vi "EMS Synchronize Status.vi"(8 "error in (no error)":errorcluster, 9 "Status":T1, 10 "error":string, 11 "Master Controller in":refnum<class "Master Controller.lvclass">) -> (0 "error out":errorcluster, 3 "Master Controller out":refnum<class "Master Controller.lvclass">)   [LabVIEW 2015, in "Master Controller Core.lvlib" / "Master Controller.lvclass"]
uses:
  Master Controller.lvclass
  SCADA Core/SCADA Abstract Messages/Simple Command Status Msg/Simple Command Status.ctl
  Communications/SCADA Communcations Actor/SCADA Communications/Controls/EMS Message Cluster.ctl
  Master Controller.lvclass/Master Controller.ctl
  Communications/SCADA Communcations Actor/SCADA Communications Messages/Transmit EMS Message Msg/Transmit EMS Message Msg.lvclass/Transmit EMS Message Msg.ctl
  <vilib>/ActorFramework/Message Enqueuer/Message Enqueuer.lvclass/Message Enqueuer.ctl
  <vilib>/ActorFramework/Message Enqueuer/Enqueue.vi
  <vilib>/ActorFramework/Message Priority Queue/Priority Enqueue.vi
  Communications/SCADA Communcations Actor/SCADA Communications Messages/Transmit EMS Message Msg/Transmit EMS Message Msg.lvclass
  Communications/SCADA Communcations Actor/SCADA Communications/SCADA Communications.lvclass
  Utilities/Message Strings.llb/Message String Utilities.lvlib
  Utilities/Status Messaging.llb/Status Messaging.lvlib
  SCADA Core/SCADA Abstract Messages/Simple Command Status Msg/Simple Command Status Msg.lvclass
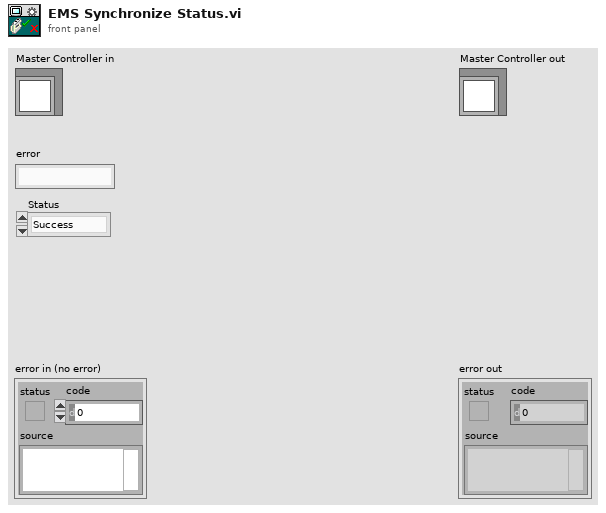
[diagram p1: front panel]
types:
  T1 = typedef "SCADA Core.lvlib/Simple Command Status Msg.lvclass/Simple Command Status.ctl" = enum16{"Success", "Failure"}
  T2 = typedef "SCADA Communcations Actor.lvlib/SCADA Communications.lvclass/EMS Message Cluster.ctl" = cluster{"Name":string, "Content":string}
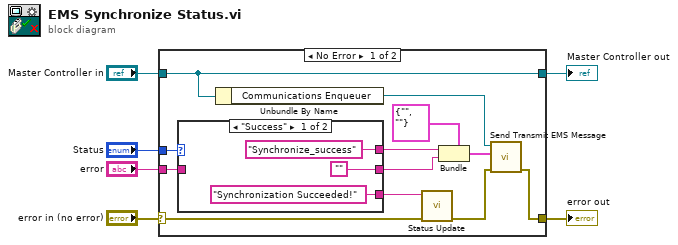
[diagram p0: block diagram]
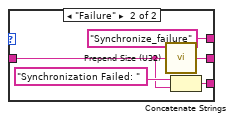
[diagram p2: hidden frame]
diagram:
  n1 = case shown="No Error" "error in (no error)" {
    selector: "error in (no error)" -> [w9 w28]
    tunnel: [w13 w28] -> w5
    tunnel: [w17 w27] -> w3
    tunnel: "Master Controller in" -> [w17 w27]
    tunnel: "error" -> [w11 _]
    tunnel: "Status" -> [w18 _]
    frame No Error {
      n2 = case shown="\"Success\"" w18 {
        tunnel: ["Synchronize_success" ("Name") "Synchronize_failure" ("Name")] -> w12
        tunnel: w11 -> [_ w23]
        tunnel: ["" w25] -> w10
        tunnel: ["Synchronization Succeeded!" w22] -> w7
        frame "Success" {
        }
        frame "Failure" {
          n3 = call "Prepend Size (U32).vi"("String in"=w23) -> ("String out"=w25:string)
          n4 = Concatenate Strings("Synchronization Failed: " ("string"), w23) -> (w22:string)
        }
      }
      n5 = Unbundle By Name(w17) -> ("Communications Enqueuer"=w15:refnum<class "Message Enqueuer.lvclass">)
      n6 = call "Status Update.vi"("error in (no error)"=w9, "Status Update"=w7) -> ("error out"=w8:errorcluster)  [unwired: 8 in, 1 out]
      n7 = Bundle(cluster=T2 {"Name"="", "Content"=""} ("Message"), "Name"=w12, "Content"=w10) -> (w14:T2)
      n8 = call "Send Transmit EMS Message.vi"("error in (no error)"=w8, "Message"=w14, "Message Enqueuer"=w15) -> ("error out"=w13:errorcluster)  [unwired: 7 in, 1 out]
    }
    frame Error {
    }
  }
  "error out" <- w5
  "Master Controller out" <- w3
